vi "1.1 Reverse Check.vi"(1 "Drive Voltage Input":fxp<+/-,20,5>) -> (0 "Drive Voltage Out":fxp<+/-,20,5>)   [LabVIEW 2010]
uses:
  <vilib>/eio/EIONode/EIONode.xnode
  <vilib>/rvi/eio/nirviEIOImplementation/nirviEIOImplementation.xnode
  <vilib>/rvi/eio/common/nirviEmuClasses.ctl
  1.0-Hindbrain Global.vi
  <vilib>/rvi/eio/common/nirviEmuTemplateMethod_noerrors.vi
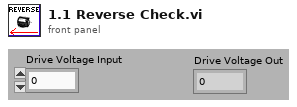
[diagram p1: front panel]
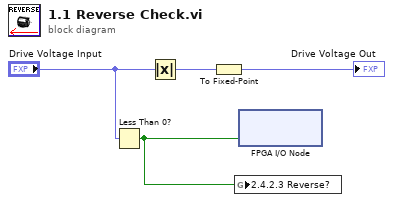
[diagram p0: block diagram]
diagram:
  n1 = Less Than 0?(x="Drive Voltage Input") -> (x < 0?=w4:bool)
  n2 = Absolute Value(x="Drive Voltage Input") -> (abs(x)=w2:fxp<+,20,5>)
  n3 = To Fixed-Point(number=w2) -> (fixed-point=→"Drive Voltage Out":fxp<+/-,20,5>)  [unwired: 1 in]
  n4 = global write "1.0-Hindbrain Global.vi" "2.4.2.3 Reverse?"(w4) -> ()
  n5 = xnode "FPGA I/O Node"("Reverse"=w4) -> ()  [unwired: 1 in, 1 out]
